vi "Autonomous Independent.vi"() -> ()   [LabVIEW 2013]
doc: "This VI is called when autonomous begins, and will automatically be terminated when autonomous ends. You can carry out timed or sensor driven robot movement independently without needing to return to the caller."
uses:
  Robot Global Data.vi
  <vilib>/Rock Robotics/WPI/RobotDrive/WPI_RobotDriveGetSetRefNum.vi
  <vilib>/Rock Robotics/WPI/RobotDrive/WPI_RobotDriveMecanumDrive_Cartesian.vi
panel:
  out "Shots Taken":i32
  out "Current Movement, for debugging":T1 {"Z Joystick Value" scale=-1.0..1.0; "Y Joystick Value" scale=1.0..-1.0; "X Joystick Value" scale=-1.0..1.0}
  in  "Array of robot movements":T2(array[cluster]) {"Z Joystick Value" scale=-1.0..1.0; "Y Joystick Value" scale=1.0..-1.0; "X Joystick Value" scale=-1.0..1.0}
  # "Be sure to right-click and choose Data Operations>>Make Current Value default if you want to save the array values with the VI"
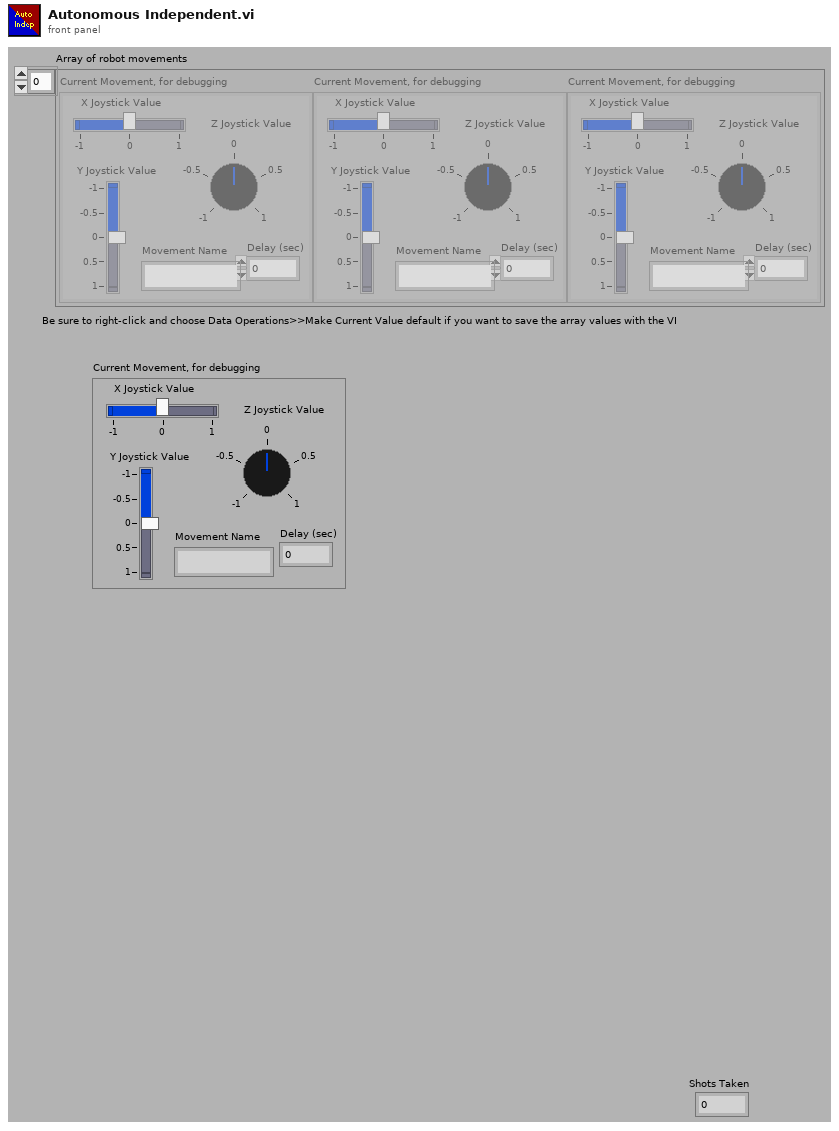
[diagram p1: front panel]
types:
  T1 = cluster{"X Joystick Value":dbl, "Y Joystick Value":dbl, "Z Joystick Value":dbl, "Delay (sec)":dbl, "Movement Name":string}
  T2 = cluster{"X Joystick Value":dbl, "Y Joystick Value":dbl, "Z Joystick Value":dbl, "Delay (sec)":dbl, "Movement Name":string}[]
  T3 = typedef "WPI_RobotDriveDevRef.ctl" = cluster{"DevStatus":errorcluster, "Motors[]":T4[], "Square Inputs":bool, "Max Output":dbl, "Isochronous":bool}
  T4 = typedef "WPI_MotorControlDeviceRef.ctl" = cluster{"DeviceStatus":errorcluster, "Type":enum16{"PWM", "CAN"}, "PWM":cluster{"Digital Module":T5, "PWM Channel":T6, "DeadBand":T7}, "CAN":cluster{"Device Number":u8, "Control Mode":T8, "Semaphore":T9, "Max Vout":dbl}, "Invert":bool, "TransformRef":T10, "InvTransformRef":T10}
  T5 = typedef "FPGA_TypedefDigitalModule.ctl" = enum16{"Digital Module 1", "Digital Module 2"}
  T6 = typedef "FPGA_DIOPWMChannel.ctl" = enum8{"PWM 1", "PWM 2", "PWM 3", "PWM 4", "PWM 5", "PWM 6", "PWM 7", "PWM 8", "PWM 9", "PWM 10", "Invalid"}
  T7 = typedef "WPI_PWMDeadband.ctl" = cluster{"Name":string, "maxPositivePwm":i32, "minPositivePwm":i32, "centerPwm":i32, "maxNegativePwm":i32, "minNegativePwm":i32, "angularRange":u16}
  T8 = typedef "WPI_CANJaguar_ControlMode.ctl" = enum8{"Percent VBus", "Current", "Speed", "Position", "Voltage"}
  T9 = typedef "Semaphore RefNum" = refnum<k1>
  T10 = typedef "WPI_PWMTransform_ConPane.ctl" = refnum<vi>
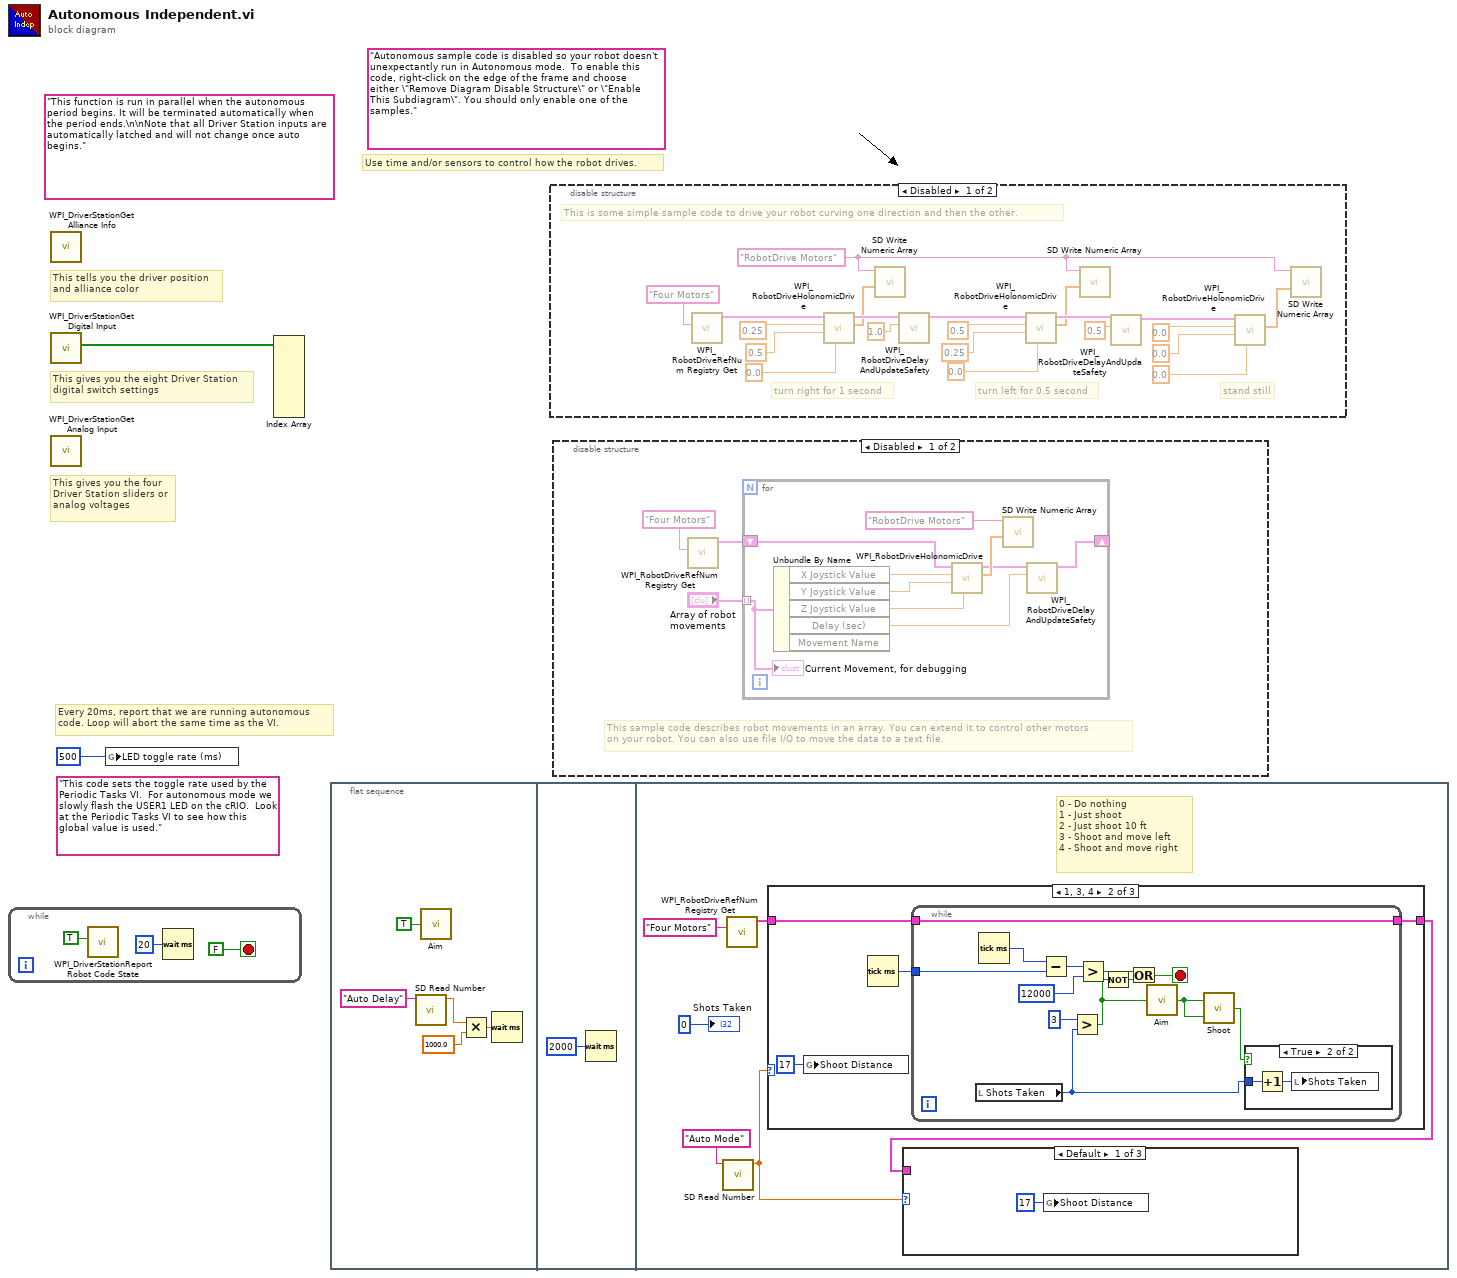
[diagram p0: block diagram]
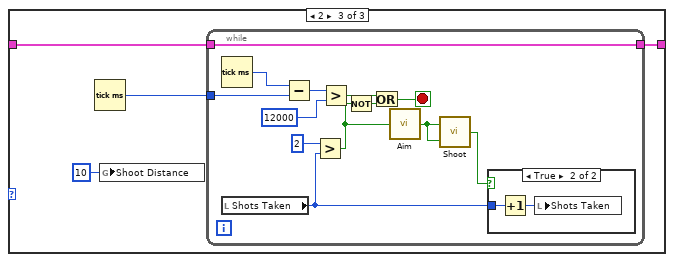
[diagram p4: hidden frame]
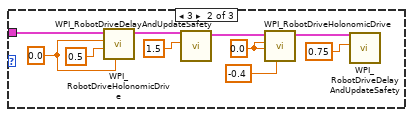
[diagram p6: hidden frame]
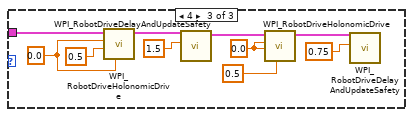
[diagram p7: hidden frame]
diagram:
  (unwired) "This code sets the toggle rate used by the Periodic Tasks VI.  For autonomous mode we slowly flash the USER1 LED on the cRIO.  Look at the Periodic Tasks VI to see how this global value is used."
  (unwired) "Autonomous sample code is disabled so your robot doesn't unexpectantly run in Autonomous mode.  To enable this code, right-click on the edge of the frame and choose either \"Remove Diagram Disable Structure\" or \"Enable This Subdiagram\". You should only enable one of the samples."
  (unwired) "This function is run in parallel when the autonomous period begins. It will be terminated automatically when the period ends.\n\nNote that all Driver Station inputs are automatically latched and will not change once auto begins."
  # "Every 20ms, report that we are running autonomous\ncode. Loop will abort the same time as the VI."
  # "Use time and/or sensors to control how the robot drives."
  # "This tells you the driver position\nand alliance color"
  # "This gives you the eight Driver Station\ndigital switch settings"
  # "This gives you the four\nDriver Station sliders or\nanalog voltages"
  n1 = while {
    stop <- FALSE stop-if-true
    n2 = call <vilib>:"WPI_DriverStationReport Robot Code State.vi"("Autonomous"=TRUE) -> ()  [unwired: 10 in, 1 out]
    n3 = Wait (ms)(milliseconds to wait=u32 20) -> ()  [unwired: 1 out]
  }
  n4 = call <vilib>:"WPI_DriverStationGet Alliance Info.vi"() -> ()  [unwired: 12 out]
  n5 = call <vilib>:"WPI_DriverStationGet Digital Input.vi"() -> ("Driver Station Digital Input (1-8)"=w2:bool[])  [unwired: 11 out]
  n6 = call <vilib>:"WPI_DriverStationGet Analog Input.vi"() -> ()  [unwired: 12 out]
  n7 = global write "Robot Global Data.vi" "LED toggle rate (ms)"(u32 500 ("LED ms toggle rate")) -> ()
  n8 = Index Array(array=w2) -> ()  [unwired: 8 in, 8 out]
  n9 = flat-sequence {
    frame #0 {
      n10 = call <vilib>:"SD Read Number.vi"("Name"="Auto Delay") -> ("Numeric"=w9:dbl)  [unwired: 8 in, 2 out]
      n11 = call "Aim.vi"("Aim"=TRUE) -> ()  [unwired: 1 out]
      n12 = Multiply(x=w9, y=1000.0) -> (x*y=w8:dbl)
      n13 = Wait (ms)(milliseconds to wait=w8) -> ()  [unwired: 1 out]
    }
    frame #1 {
      n14 = Wait (ms)(milliseconds to wait=u32 2000) -> ()  [unwired: 1 out]
    }
    frame #2 {
      # "0 - Do nothing\n1 - Just shoot\n2 - Just shoot 10 ft\n3 - Shoot and move left\n4 - Shoot and move right"
      n15 = call <vilib>:"SD Read Number.vi"("Name"="Auto Mode") -> ("Numeric"=w13:dbl)  [unwired: 8 in, 2 out]
      n16 = call <vilib>:"WPI_RobotDriveRefNum Registry Get.vi"("refnum name"="Four Motors") -> ("RobotDriveDevRef"=w14:T3)  [unwired: 1 in, 9 out]
      n17 = case shown="1, 3, 4" w13 {
        tunnel: [w18 w20 w39] -> w16
        tunnel: w14 -> [w18 w21 w40]
        frame 0, Default {
        }
        frame 1, 3, 4 {
          n18 = global write "Robot Global Data.vi" "Shoot Distance"(17 ("Shoot Distance")) -> ()
          n19 = Tick Count (ms)() -> (millisecond timer value=w22:u32)
          n20 = while {
            tunnel: w21 -> [w32]
            tunnel: [w32] -> w20
            tunnel: w22 -> [w26]
            stop <- w27 stop-if-true
            n21 = local read "Shots Taken"() -> (w35:i32)
            n22 = Tick Count (ms)() -> (millisecond timer value=w25:u32)
            n23 = Subtract(x=w25, y=w26) -> (x-y=w31:u32)
            n24 = Greater?(x=3, y=w35) -> (0:w28:bool)
            n25 = Greater?(x=w31, y=u32 12000) -> (0:w29:bool)
            n26 = Not(x=w28) -> (.not. x?=w24:bool)
            n27 = Or(x=w29, y=w24) -> (x .or. y?=w27:bool)
            n28 = call "Aim.vi"("Aim"=w28) -> ("Ready"=w33:bool)
            n29 = call "Shoot.vi"("Shoot"=w33, "Aiming"=w33) -> ("Done"=w34:bool)
            n30 = case shown="True" w34 {
              tunnel: w35 -> [_ w36]
              frame False {
              }
              frame True {
                n31 = Increment(x=w36) -> (x+1=w37:i32)
                n32 = local write "Shots Taken"(w37) -> ()
              }
            }
          }
        }
        frame 2 {
          n33 = Tick Count (ms)() -> (millisecond timer value=w41:u32)
          n34 = global write "Robot Global Data.vi" "Shoot Distance"(10 ("Shoot Distance")) -> ()
          n35 = while {
            tunnel: w40 -> [w51]
            tunnel: [w51] -> w39
            tunnel: w41 -> [w45]
            stop <- w46 stop-if-true
            n36 = Tick Count (ms)() -> (millisecond timer value=w44:u32)
            n37 = local read "Shots Taken"() -> (w54:i32)
            n38 = Subtract(x=w44, y=w45) -> (x-y=w50:u32)
            n39 = Greater?(x=2, y=w54) -> (0:w47:bool)
            n40 = Greater?(x=w50, y=u32 12000) -> (0:w48:bool)
            n41 = Not(x=w47) -> (.not. x?=w43:bool)
            n42 = Or(x=w48, y=w43) -> (x .or. y?=w46:bool)
            n43 = call "Aim.vi"("Aim"=w47) -> ("Ready"=w52:bool)
            n44 = call "Shoot.vi"("Shoot"=w52, "Aiming"=w52) -> ("Done"=w53:bool)
            n45 = case shown="True" w53 {
              tunnel: w54 -> [_ w55]
              frame False {
              }
              frame True {
                n46 = Increment(x=w55) -> (x+1=w56:i32)
                n47 = local write "Shots Taken"(w56) -> ()
              }
            }
          }
        }
      }
      n48 = case shown="Default" w13 {
        tunnel: w16 -> [_ w66 w68]
        frame Default {
          n49 = global write "Robot Global Data.vi" "Shoot Distance"(17 ("Shoot Distance")) -> ()
        }
        frame 3 {
          w62 = 0.0 ("X axis value")
          w61 = 0.0 ("X axis value")
          n50 = call-poly <vilib>:"WPI_RobotDriveHolonomicDrive.vi"("Rotation"=w61, "Y"=0.5 ("X axis value"), "X"=w61, "RobotDriveDevRef"=w66) -> ("RobotDriveDevRef"=w67:T3)  [unwired: 5 in, 2 out]
          n51 = call <vilib>:"WPI_RobotDriveDelayAndUpdateSafety.vi"("Delay (s)"=1.5, "RobotDriveDevRef"=w67) -> ("RobotDriveDevRef 2"=w63:T3)  [unwired: 8 in, 1 out]
          n52 = call-poly <vilib>:"WPI_RobotDriveHolonomicDrive.vi"("Rotation"=-0.4, "Y"=w62, "X"=w62, "RobotDriveDevRef"=w63) -> ("RobotDriveDevRef"=w65:T3)  [unwired: 5 in, 2 out]
          n53 = call <vilib>:"WPI_RobotDriveDelayAndUpdateSafety.vi"("Delay (s)"=0.75, "RobotDriveDevRef"=w65) -> ()  [unwired: 8 in, 2 out]
        }
        frame 4 {
          w73 = 0.0 ("X axis value")
          w74 = 0.0 ("X axis value")
          n54 = call-poly <vilib>:"WPI_RobotDriveHolonomicDrive.vi"("Rotation"=w74, "Y"=0.5 ("X axis value"), "X"=w74, "RobotDriveDevRef"=w68) -> ("RobotDriveDevRef"=w69:T3)  [unwired: 5 in, 2 out]
          n55 = call <vilib>:"WPI_RobotDriveDelayAndUpdateSafety.vi"("Delay (s)"=1.5, "RobotDriveDevRef"=w69) -> ("RobotDriveDevRef 2"=w72:T3)  [unwired: 8 in, 1 out]
          n56 = call-poly <vilib>:"WPI_RobotDriveHolonomicDrive.vi"("Rotation"=0.5, "Y"=w73, "X"=w73, "RobotDriveDevRef"=w72) -> ("RobotDriveDevRef"=w70:T3)  [unwired: 5 in, 2 out]
          n57 = call <vilib>:"WPI_RobotDriveDelayAndUpdateSafety.vi"("Delay (s)"=0.75, "RobotDriveDevRef"=w70) -> ()  [unwired: 8 in, 2 out]
        }
      }
      "Shots Taken" <- 0 ("Shots Taken")
    }
  }
  n58 = disable-structure shown="Disabled" {
    frame Disabled {
      w81 = "RobotDrive Motors" ("Name")
      # "This is some simple sample code to drive your robot curving one direction and then the other."
      # "stand still"
      # "turn left for 0.5 second"
      # "turn right for 1 second"
      n59 = call <vilib>:"WPI_RobotDriveRefNum Registry Get.vi"("refnum name"="Four Motors") -> ("RobotDriveDevRef"=w85:T3)  [unwired: 1 in, 9 out]
      n60 = call-poly <vilib>:"WPI_RobotDriveHolonomicDrive.vi"("Rotation"=0.0, "Y"=0.5 ("X axis value"), "X"=0.25 ("X axis value"), "RobotDriveDevRef"=w85) -> ("Motor Values"=w84:dbl[], "RobotDriveDevRef"=w92:T3)  [unwired: 5 in, 1 out]
      n61 = call <vilib>:"SD Write Numeric Array.vi"("Numeric Array"=w84, "Name"=w81) -> ()  [unwired: 8 in, 2 out]
      n62 = call <vilib>:"WPI_RobotDriveDelayAndUpdateSafety.vi"("Delay (s)"=1.0, "RobotDriveDevRef"=w92) -> ("RobotDriveDevRef 2"=w91:T3)  [unwired: 8 in, 1 out]
      n63 = call-poly <vilib>:"WPI_RobotDriveHolonomicDrive.vi"("Rotation"=0.0, "Y"=0.25 ("X axis value"), "X"=0.5 ("X axis value"), "RobotDriveDevRef"=w91) -> ("Motor Values"=w83:dbl[], "RobotDriveDevRef"=w90:T3)  [unwired: 5 in, 1 out]
      n64 = call <vilib>:"SD Write Numeric Array.vi"("Numeric Array"=w83, "Name"=w81) -> ()  [unwired: 8 in, 2 out]
      n65 = call <vilib>:"WPI_RobotDriveDelayAndUpdateSafety.vi"("Delay (s)"=0.5, "RobotDriveDevRef"=w90) -> ("RobotDriveDevRef 2"=w89:T3)  [unwired: 8 in, 1 out]
      n66 = call-poly <vilib>:"WPI_RobotDriveHolonomicDrive.vi"("Rotation"=0.0 ("X axis value"), "Y"=0.0 ("X axis value"), "X"=0.0 ("X axis value"), "RobotDriveDevRef"=w89) -> ("Motor Values"=w82:dbl[])  [unwired: 5 in, 2 out]
      n67 = call <vilib>:"SD Write Numeric Array.vi"("Numeric Array"=w82, "Name"=w81) -> ()  [unwired: 8 in, 2 out]
    }
    frame Enabled {
    }
  }
  n68 = disable-structure shown="Disabled" {
    frame Disabled {
      # "This sample code describes robot movements in an array. You can extend it to control other motors\non your robot. You can also use file I/O to move the data to a text file."
      n69 = call <vilib>:"WPI_RobotDriveRefNum Registry Get.vi"("refnum name"="Four Motors") -> ("RobotDriveDevRef"=w100:T3)  [unwired: 1 in, 9 out]
      n70 = for {
        shift-right: [w107] -> _
        shift-left: w100 -> [w108]
        tunnel: "Array of robot movements" -> [w103] mode=indexing
        n71 = Unbundle By Name(w103) -> ("X Joystick Value"=w106:dbl, "Y Joystick Value"=w105:dbl, "Z Joystick Value"=w102:dbl, "Delay (sec)"=w104:dbl)  [unwired: 1 out]
        n72 = call-poly <vilib>:"WPI_RobotDriveHolonomicDrive.vi"("Rotation"=w102, "Y"=w105, "X"=w106, "RobotDriveDevRef"=w108) -> ("Motor Values"=w110:dbl[], "RobotDriveDevRef"=w109:T3)  [unwired: 5 in, 1 out]
        n73 = call <vilib>:"SD Write Numeric Array.vi"("Numeric Array"=w110, "Name"="RobotDrive Motors") -> ()  [unwired: 8 in, 2 out]
        n74 = call <vilib>:"WPI_RobotDriveDelayAndUpdateSafety.vi"("Delay (s)"=w104, "RobotDriveDevRef"=w109) -> ("RobotDriveDevRef 2"=w107:T3)  [unwired: 8 in, 1 out]
        "Current Movement, for debugging" <- w103
      }
    }
    frame Enabled {
    }
  }
